vi "FGV SingleCode.vi"() -> ()   [LabVIEW 2022 SP3]
panel:
  out "Data Output 2":dbl
  out "Data Output":dbl
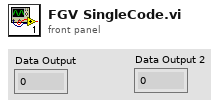
[diagram p1: front panel]
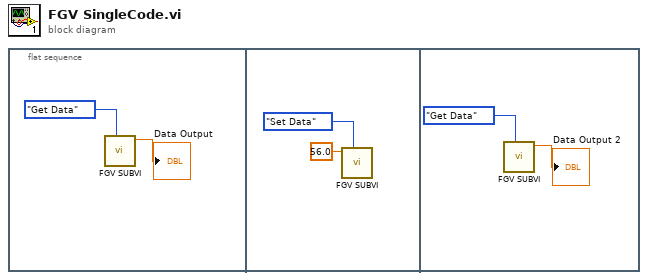
[diagram p0: block diagram]
diagram:
  n1 = flat-sequence {
    frame #0 {
      n2 = call "FGV SUBVI.vi"("Enum"=enum16{"Get Data", "Set Data"}."Get Data") -> ("Data Input out"=→"Data Output":dbl)  [unwired: 10 in]
    }
    frame #1 {
      n3 = call "FGV SUBVI.vi"("Enum"=enum16{"Get Data", "Set Data"}."Set Data", "Data Input in"=56.0) -> ()  [unwired: 9 in, 1 out]
    }
    frame #2 {
      n4 = call "FGV SUBVI.vi"("Enum"=enum16{"Get Data", "Set Data"}."Get Data") -> ("Data Input out"=→"Data Output 2":dbl)  [unwired: 10 in]
    }
  }
